vi "RSNRPZ Send Software Trigger.vi"(8 "error in (no error)":errorcluster, 10 "Channel (1)":i32=1, 11 "VISA session":refnum<visa-resource-name> caption="VISA resource name") -> (0 "error out":errorcluster, 3 "dup VISA session":refnum<visa-resource-name> caption="VISA resource name")   [LabVIEW 2010]
doc: "Triggers a BUS event. If the sensor is in the WAIT_FOR_TRG state and the source for the trigger source is set to BUS, the sensor enters the MEASURING state. This VI invalidates all current measuring results. A query of measurement data following this VI will thus always return the measured value determined in response to this VI.\n\nRemote-control command(s):\n*TRG"
uses:
  rsnrpz_32.dll
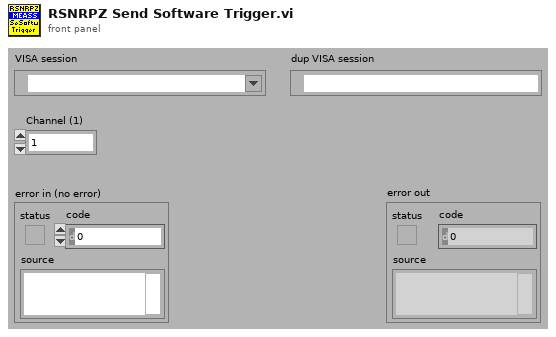
[diagram p1: front panel]
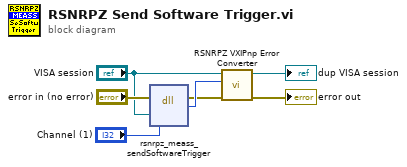
[diagram p0: block diagram]
diagram:
  n1 = dll-call lib="rsnrpz_32.dll" fn="rsnrpz_meass_sendSoftwareTrigger"(error in="error in (no error)", "VISA Session"="VISA session", "Channel"="Channel (1)") -> (error out=w5:errorcluster, "Status"=w7:i32)  [unwired: 4 in, 1 out]
  n2 = call <instrlib>:"RSNRPZ VXIPnp Error Converter.vi"("error in"=w5, "VXIPnp error code"=w7, "VISA session"="VISA session") -> ("error out"=→"error out":errorcluster, "dup VISA session"=→"dup VISA session":refnum<visa-resource-name>)  [unwired: 7 in]
